vi "WritingDataFile Message Loop.vi"(8 "error in (no error)":errorcluster, 11 "Message Queues":T1) -> (0 "error out":errorcluster)   [LabVIEW 2020, in "WritingDataFile.lvlib"]
uses:
  WritingDataFile.lvlib
  support/Message Queue/All Message Queues.ctl
  support/Message Queue/Message Cluster.ctl
  Modbus/Modbus PLC Data All.ctl
  Modbus/Modbus FVIR Control.ctl
  Modbus/Modbus LDO Control.ctl
  Data to Save.ctl
  <vilib>/Utility/file.llb/Write Delimited Spreadsheet (string).vi
  support/Message Queue/Enqueue Message (Single).vi
  support/Message Queue/Message Queue.lvlib
  Logging/Logging.lvlib
  HeaderForCSV.ctl
  HeaderForCSV_LDO.ctl
panel:
  out "Start time LDO":string
  out "Start time FVIR":string
  out "Numeric":i32
  out "Loop counter":i32
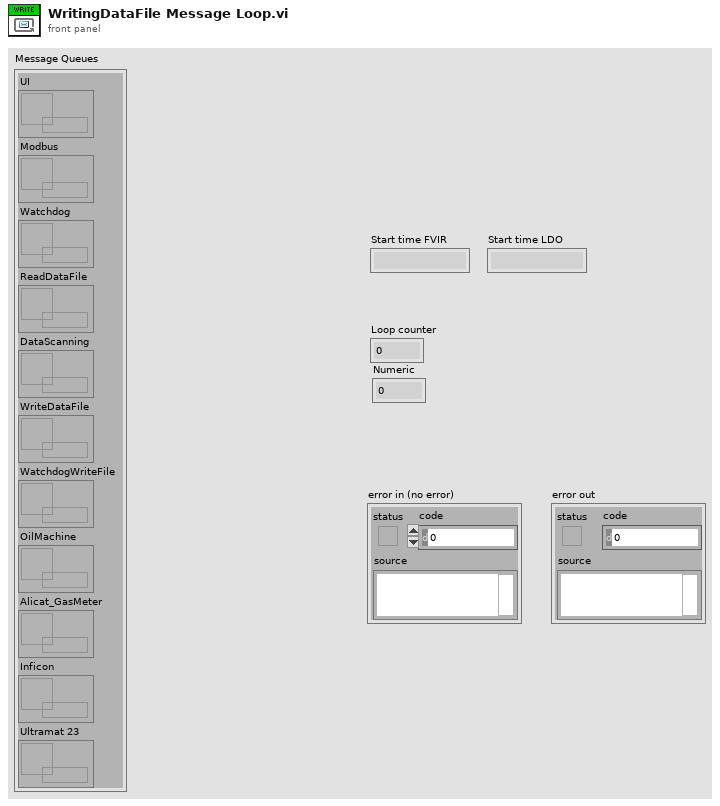
[diagram p1: front panel]
types:
  T1 = typedef "Message Queue.lvlib/All Message Queues.ctl" = cluster{"UI":refnum<queue>, "Modbus":refnum<queue>, "Watchdog":refnum<queue>, "ReadDataFile":refnum<queue>, "DataScanning":refnum<queue>, "WriteDataFile":refnum<queue>, "WatchdogWriteFile":refnum<queue>, "OilMachine":refnum<queue>, "Alicat_GasMeter":refnum<queue>, "Inficon":refnum<queue>, "Ultramat 23":refnum<queue>}
  T2 = typedef "Modbus PLC Data All.ctl" = cluster{"FVIR Data Input":T3, "LDO Control Input":T4, "PLC Input Registers":i16[], "Data to Save":T5}
  T3 = typedef "Modbus FVIR Control.ctl" = cluster{"Spare 15":bool, "Spare 14":bool, "Actuator mannequin is going to Work Pos - FVIR":bool, "Actuator mannequin is going to Home Pos - FVIR":bool, "Test chamber is in sequence - FVIR ":bool, "Water flow DRK375 is open - FVIR":bool, "Gas Solenoid Valve - FVIR":bool, "Water Inlet Valve - FVIR":bool, "Water Outlet Flow Proportional - FVIR":bool, "Start recording data - FVIR":bool, "Actuator spill can is going to Work Pos - FVIR":bool, "Actuator spill can is going to Home Pos - FVIR":bool, "Water Outlet Valve - FVIR":bool, "Can is spilling - FVIR":bool, "Mannequin is moving - FVIR":bool, "FVIR PLC lifebit":bool, "Status for Error - FVIR":string, "Error-FVIR":bool, "Sensors -FVIR":string[][]}
  T4 = typedef "Modbus LDO Control.ctl" = cluster{"LDO PLC Life Bit":bool, "Start recording data - LDO":bool, "Spare 1":bool, "Water Outlet Valve - LDO":bool, "Water Inlet Valve - LDO":bool, "Gas Solenoid Valve - LDO":bool, "Water flow DRK375 is open - LDO":bool, "Test chamber is in sequence - LDO":bool, "Oil spray 0.8cc/min - LDO":bool, "Oil spray 1.1cc/min - LDO":bool, "Oil spray 1.33cc/min - LDO":bool, "Rotary Actuator (ON/OFF) - LDO":bool, "Water Outlet Flow Proportional - LDO":bool, "Conveyor ON/OFF":bool, "Blower ON/OFF":bool, "Spare 4":bool, "Status for error - LDO":string, "Error - LDO":bool, "Sensor Data":string[][], "Thermal Efficiency Rate (GPM)":dbl, "Thermal Efficiency":dbl, "Totalized Flow (Gallons)":dbl, "Counter of oil injections 1.33 cc/min":u16, "Counter of burner cycle":u16, "Counter of oil injections 1.1 cc/min":u16, "Counter of oil injections 0.8 cc/min":u16, "Previous Totalizer (Gallons)":dbl, "Gallon Adder Input":dbl}
  T5 = typedef "Data to Save.ctl" = cluster{"LDO Full Data":string[][], "FVIR Full Data":string[][], "Test Case - FVIR":string, "Test Case - LDO":string}
  T6 = typedef "WritingDataFile.lvlib/HeaderForCSV.ctl" = string[]
  T7 = typedef "WritingDataFile.lvlib/HeaderForCSV_LDO.ctl" = string[]
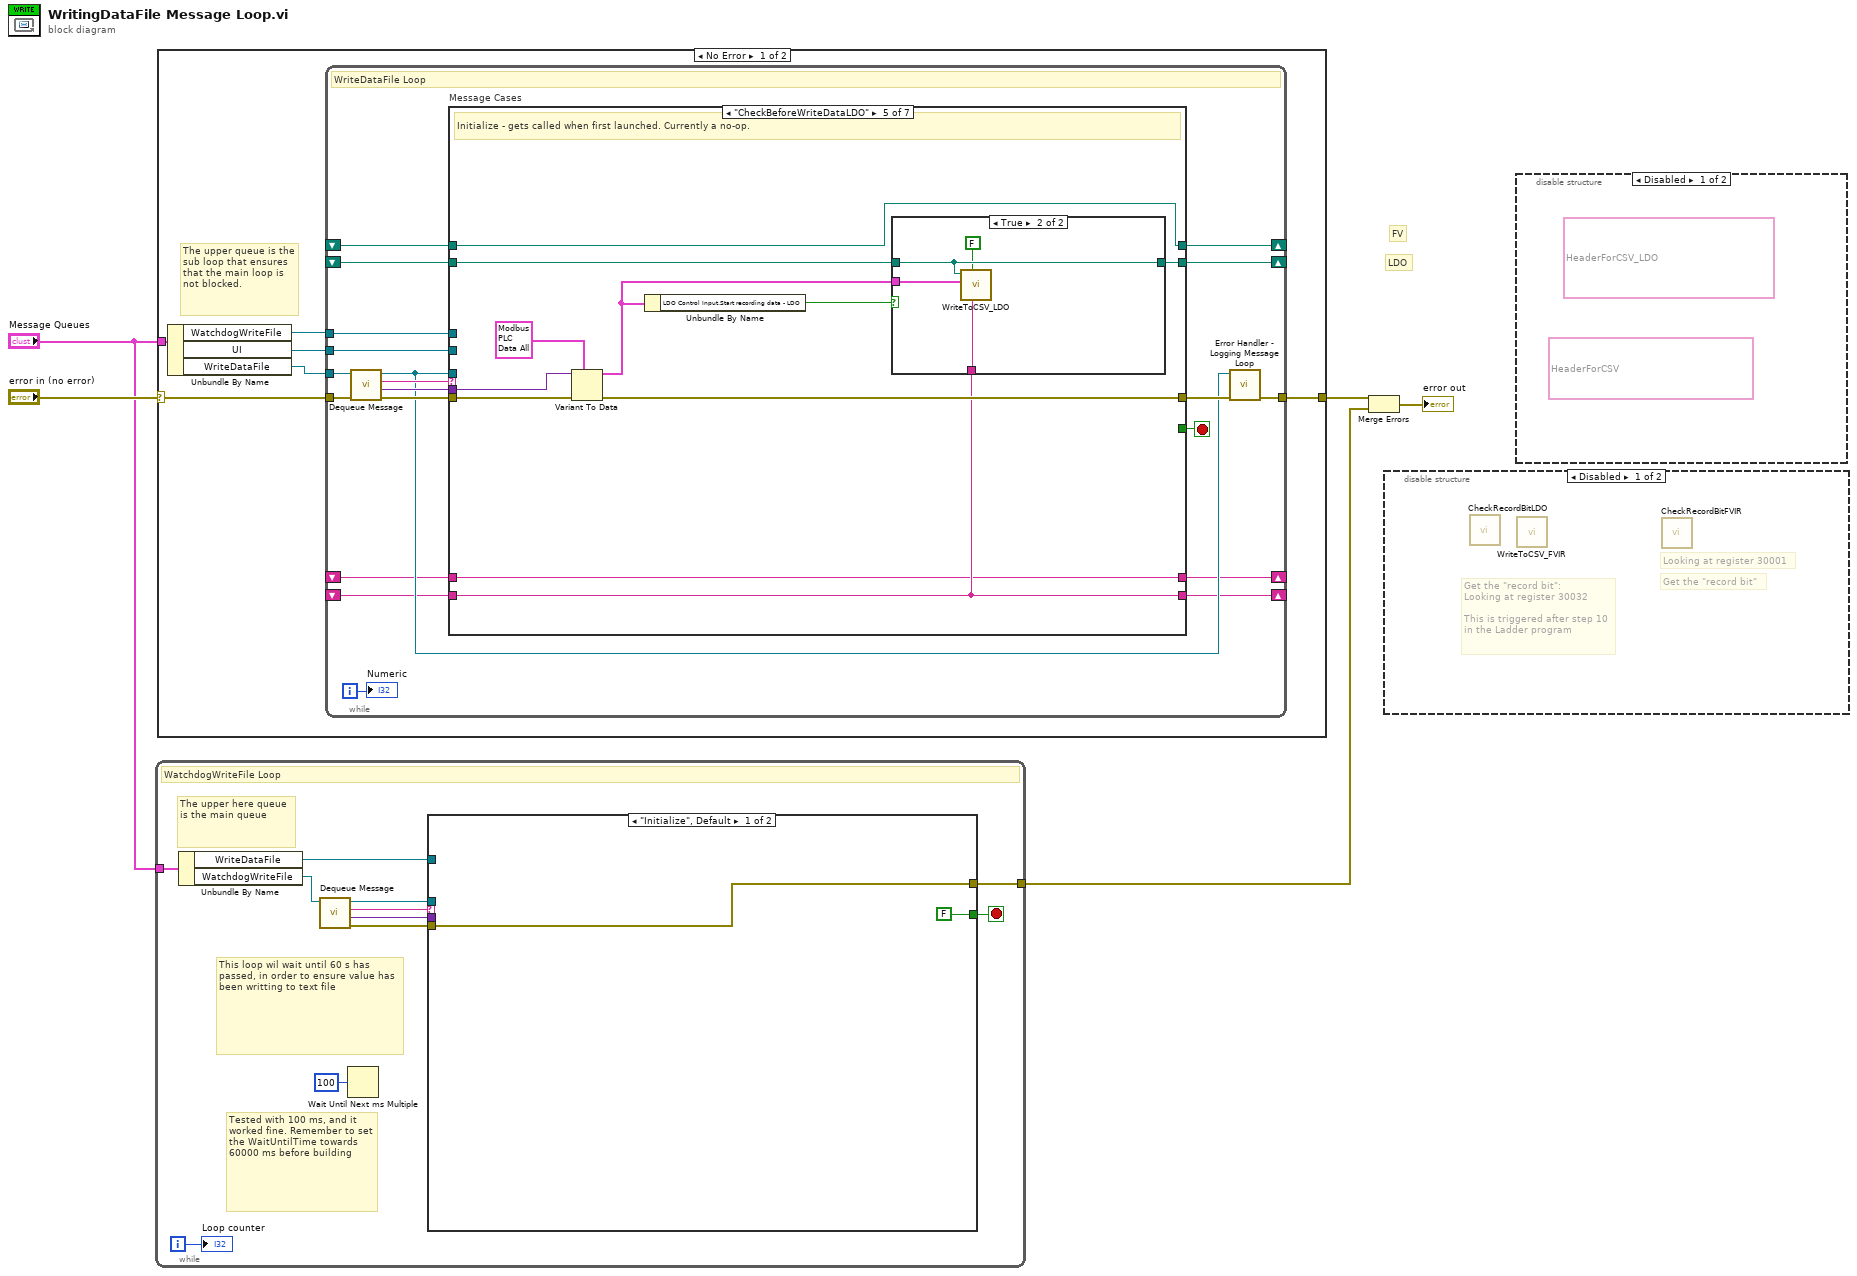
[diagram p0: block diagram]
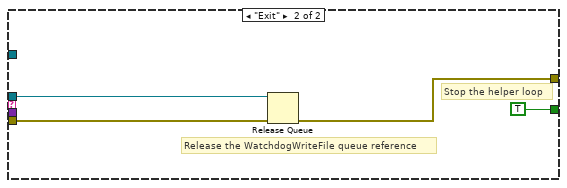
[diagram p4: hidden frame]
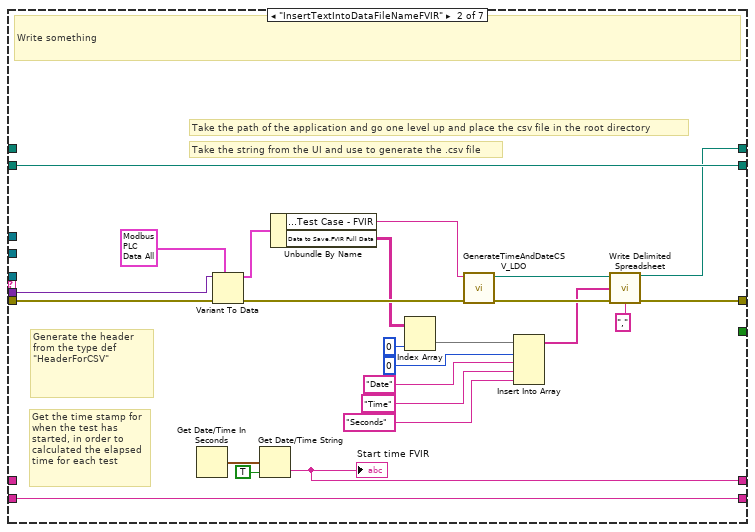
[diagram p6: hidden frame]
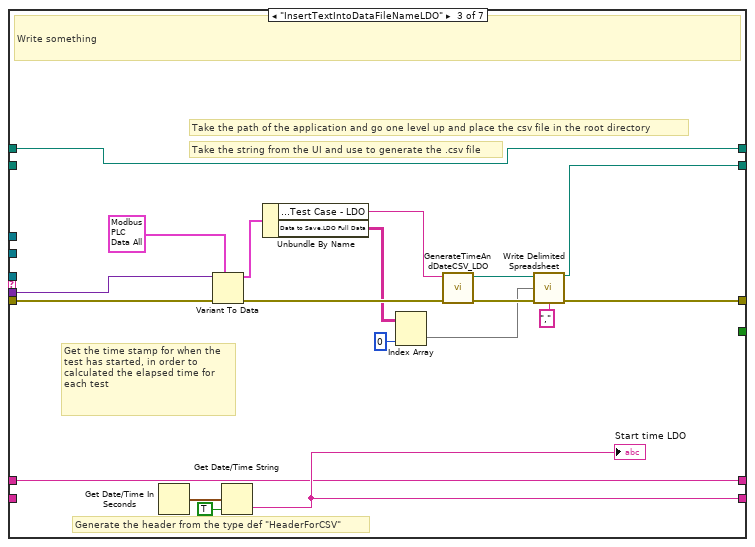
[diagram p7: hidden frame]
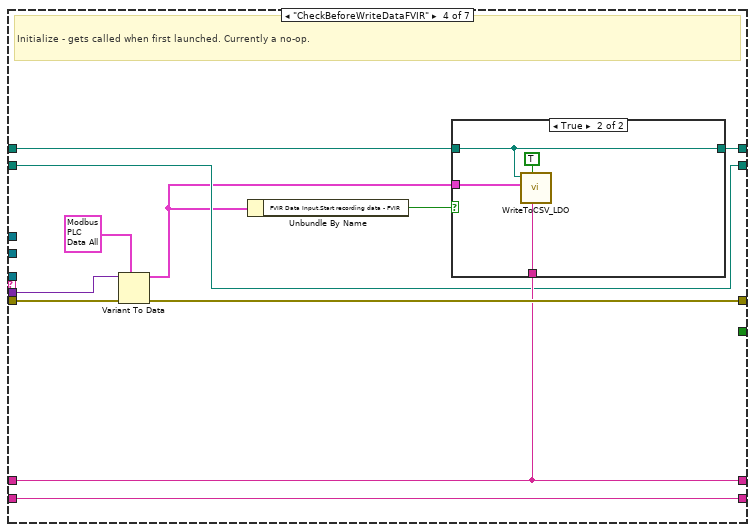
[diagram p8: hidden frame]
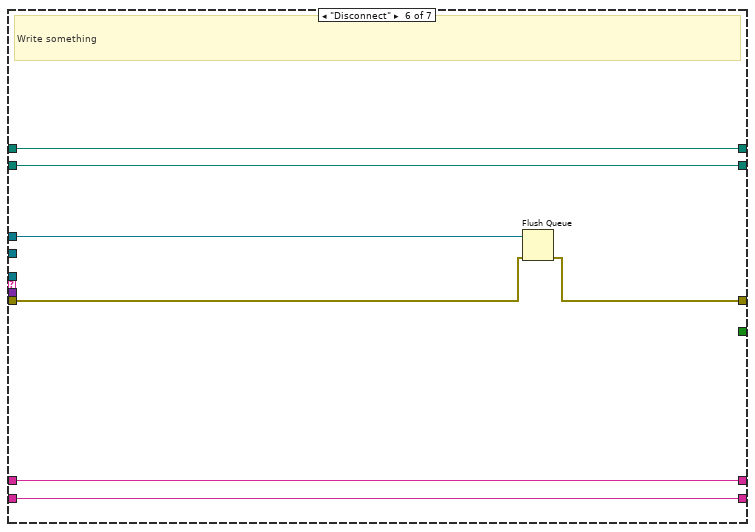
[diagram p11: hidden frame]
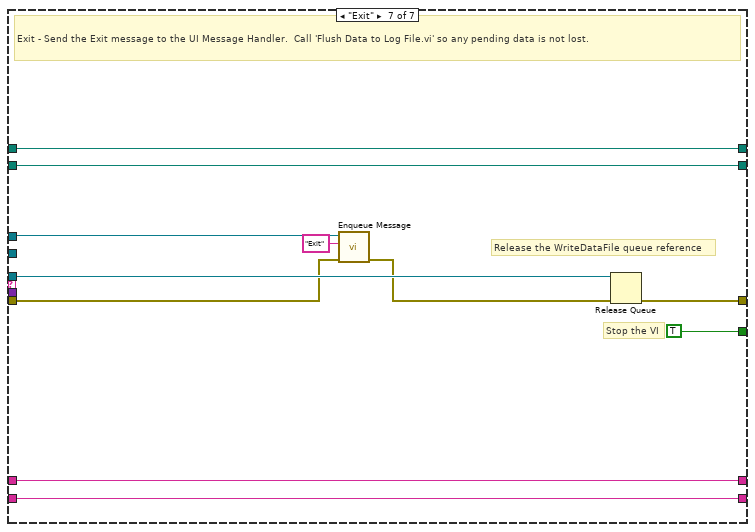
[diagram p12: hidden frame]
diagram:
  # "LDO"
  # "FV"
  n1 = while {
    tunnel: "Message Queues" -> [w16]
    tunnel: [w12] -> w2
    i -> [w7]
    stop <- w13 stop-if-true
    # "Tested with 100 ms, and it worked fine. Remember to set the WaitUntilTime towards 60000 ms before building"
    # "The upper here queue is the main queue"
    # "This loop wil wait until 60 s has passed, in order to ensure value has been writting to text file"
    # "WatchdogWriteFile Loop"
    n2 = Unbundle By Name(w16) -> ("WriteDataFile"=w10:refnum<queue>, "WatchdogWriteFile"=w11:refnum<queue>)
    n3 = call "Dequeue Message.vi"("Message Queue"=w11) -> ("error out"=w14:errorcluster, "Message Data"=w6:variant, "Message"=w15:string, "dup Message Queue"=w9:refnum<queue>)  [unwired: 7 in]
    n4 = Wait Until Next ms Multiple(millisecond multiple=u32 100) -> ()  [unwired: 1 out]
    n5 = case shown="\"Initialize\", Default" w15 {
      tunnel: w14 -> [w18 w22]
      tunnel: [w18 w21] -> w12
      tunnel: [FALSE TRUE] -> w13
      tunnel: w10 -> [_ _]
      tunnel: w9 -> [_ w19]
      tunnel: w6 -> [_ _]
      frame "Initialize", Default {
      }
      frame "Exit" {
        # "Release the WatchdogWriteFile queue reference"
        # "Stop the helper loop"
        n6 = Release Queue(queue=w19, error in (no error)=w22) -> (error out=w21:errorcluster)  [unwired: 1 in, 2 out]
      }
    }
    "Loop counter" <- w7
  }
  n7 = case shown="No Error" "error in (no error)" {
    selector: "error in (no error)" -> [w26 w147]
    tunnel: "Message Queues" -> [w28 _]
    tunnel: [w27 w147] -> w3
    frame No Error {
      # "The upper queue is the sub loop that ensures that the main loop is not blocked."
      n8 = Unbundle By Name(w28) -> ("WatchdogWriteFile"=w25:refnum<queue>, "UI"=w23:refnum<queue>, "WriteDataFile"=w24:refnum<queue>)
      n9 = while {
        tunnel: w24 -> [w43]
        tunnel: w25 -> [w40]
        tunnel: w26 -> [w47]
        tunnel: [w42] -> w27
        tunnel: w23 -> [w38]
        shift-right: [w36] -> _
        shift-left: _ -> [w35]
        shift-right: [w34] -> _
        shift-left: _ -> [w33]
        shift-right: [w32] -> _
        shift-left: _ -> [w31]
        shift-right: [w30] -> _
        shift-left: _ -> [w29]
        i -> [w37]
        stop <- w48 stop-if-true
        # "WriteDataFile Loop"
        n10 = call "Dequeue Message.vi"("error in (no error)"=w47, "Message Queue"=w43) -> ("error out"=w46:errorcluster, "Message Data"=w44:variant, "Message"=w45:string, "dup Message Queue"=w39:refnum<queue>)  [unwired: 6 in]
        n11 = case "Message Cases" shown="\"CheckBeforeWriteDataLDO\"" w45 {
          tunnel: w39 -> [_ _ _ _ _ _ w145]
          tunnel: w46 -> [w53 w77 w96 w107 w123 w134 w140]
          tunnel: [w53 w66 w85 w105 w121 w133 w144] -> w41
          tunnel: [_ _ _ _ _ _ TRUE] -> w48
          tunnel: w44 -> [_ w76 w95 w106 w122 _ _]
          tunnel: w40 -> [_ _ _ _ _ w135 w143]
          tunnel: w38 -> [_ _ _ _ _ _ _]
          tunnel: [w49 w71 w84 w100 w118 w129 w136] -> w36
          tunnel: w35 -> [w49 w71 _ w100 w119 w129 w136]
          tunnel: [w52 w73 w90 w104 w117 w132 w139] -> w34
          tunnel: w33 -> [w52 _ w90 w104 w117 w132 w139]
          tunnel: [w50 w65 w89 w103 w116 w130 w137] -> w32
          tunnel: w31 -> [w50 _ w89 w102 w116 w130 w137]
          tunnel: [w51 w72 w91 w101 w120 w131 w138] -> w30
          tunnel: w29 -> [w51 w72 _ w101 w120 w131 w138]
          frame "Initialize", Default {
            # "Initialize - gets called when first launched. Currently a no-op."
          }
          frame "InsertTextIntoDataFileNameFVIR" {
            # "Get the time stamp for when the test has started, in order to calculated the elapsed time for each test"
            # "Generate the header from the type def \"HeaderForCSV\""
            # "Take the string from the UI and use to generate the .csv file"
            # "Take the path of the application and go one level up and place the csv file in the root directory"
            # "Write something"
            n12 = Get Date/Time In Seconds() -> (seconds since 1Jan1904=w75:timestamp)
            n13 = Variant To Data(error in=w77, type=T2 {"FVIR Data Input"={"Spare 15"=FALSE, "Spare 14"=FALSE, "Actuator mannequin is going to Work Pos - FVIR"=FALSE, "Actuator mannequin is going to Home Pos - FVIR"=FALSE, "Test chamber is in sequence - FVIR "=FALSE, "Water flow DRK375 is open - FVIR"=FALSE, "Gas Solenoid Valve - FVIR"=FALSE, "Water Inlet Valve - FVIR"=FALSE, "Water Outlet Flow Proportional - FVIR"=FALSE, "Start recording data - FVIR"=FALSE, "Actuator spill can is going to Work Pos - FVIR"=FALSE, "Actuator spill can is going to Home Pos - FVIR"=FALSE, "Water Outlet Valve - FVIR"=FALSE, "Can is spilling - FVIR"=FALSE, "Mannequin is moving - FVIR"=FALSE, "FVIR PLC lifebit"=FALSE, "Status for Error - FVIR"="", "Error-FVIR"=FALSE, "Sensors -FVIR"=[]}, "LDO Control Input"={"LDO PLC Life Bit"=FALSE, "Start recording data - LDO"=FALSE, "Spare 1"=FALSE, "Water Outlet Valve - LDO"=FALSE, "Water Inlet Valve - LDO"=FALSE, "Gas Solenoid Valve - LDO"=FALSE, "Water flow DRK375 is open - LDO"=FALSE, "Test chamber is in sequence - LDO"=FALSE, "Oil spray 0.8cc/min - LDO"=FALSE, "Oil spray 1.1cc/min - LDO"=FALSE, "Oil spray 1.33cc/min - LDO"=FALSE, "Rotary Actuator (ON/OFF) - LDO"=FALSE, "Water Outlet Flow Proportional - LDO"=FALSE, "Conveyor ON/OFF"=FALSE, "Blower ON/OFF"=FALSE, "Spare 4"=FALSE, "Status for error - LDO"="", "Error - LDO"=FALSE, "Sensor Data"=[], "Thermal Efficiency Rate (GPM)"=0.0, "Thermal Efficiency"=0.0, "Totalized Flow (Gallons)"=0.0, "Counter of oil injections 1.33 cc/min"=0, "Counter of burner cycle"=0, "Counter of oil injections 1.1 cc/min"=0, "Counter of oil injections 0.8 cc/min"=0, "Previous Totalizer (Gallons)"=0.0, "Gallon Adder Input"=0.0}, "PLC Input Registers"=[], "Data to Save"={"LDO Full Data"=[], "FVIR Full Data"=[], "Test Case - FVIR"="", "Test Case - LDO"=""}} ("PLC Data Out"), Variant=w76) -> (data=w64:T2, error out=w69:errorcluster)
            n14 = Get Date/Time String(seconds (now)=w75, want seconds? (F)=TRUE) -> (time string=w73:string)  [unwired: 1 in, 1 out]
            "Start time FVIR" <- w73
            n15 = Unbundle By Name(w64) -> ("Data to Save.Test Case - FVIR"=w63:string, "Data to Save.FVIR Full Data"=w58:string[][])
            n16 = Index Array(array=w58, index (col)=0 ("disabled index (col)")) -> (element=w62:string[])  [unwired: 1 in]
            n17 = call "GenerateTimeAndDateCSV_LDO.vi"("error in (no error)"=w69, "Test string input"=w63) -> ("error out"=w67:errorcluster, "path for csv file"=w68:path)  [unwired: 8 in]
            n18 = Insert Into Array(array=w62, index=0, new element #1="Date" ("new element/subarray"), new element #2="Time" ("new element/subarray"), new element #3="Seconds" ("new element/subarray")) -> (w57:string[])
            n19 = call-poly <vilib>:"Write Delimited Spreadsheet.vi"("file path (dialog if empty)"=w68, "1D data"=w57, "error in (no error)"=w67, "delimiter (\\t)"="," ("delimiter (\\t)")) -> ("new file path (Not A Path if cancelled)"=w65:path, "error out"=w66:errorcluster)  [unwired: 10 in]
          }
          frame "InsertTextIntoDataFileNameLDO" {
            # "Get the time stamp for when the test has started, in order to calculated the elapsed time for each test"
            # "Generate the header from the type def \"HeaderForCSV\""
            # "Take the string from the UI and use to generate the .csv file"
            # "Take the path of the application and go one level up and place the csv file in the root directory"
            # "Write something"
            n20 = Get Date/Time In Seconds() -> (seconds since 1Jan1904=w94:timestamp)
            n21 = Variant To Data(error in=w96, type=T2 {"FVIR Data Input"={"Spare 15"=FALSE, "Spare 14"=FALSE, "Actuator mannequin is going to Work Pos - FVIR"=FALSE, "Actuator mannequin is going to Home Pos - FVIR"=FALSE, "Test chamber is in sequence - FVIR "=FALSE, "Water flow DRK375 is open - FVIR"=FALSE, "Gas Solenoid Valve - FVIR"=FALSE, "Water Inlet Valve - FVIR"=FALSE, "Water Outlet Flow Proportional - FVIR"=FALSE, "Start recording data - FVIR"=FALSE, "Actuator spill can is going to Work Pos - FVIR"=FALSE, "Actuator spill can is going to Home Pos - FVIR"=FALSE, "Water Outlet Valve - FVIR"=FALSE, "Can is spilling - FVIR"=FALSE, "Mannequin is moving - FVIR"=FALSE, "FVIR PLC lifebit"=FALSE, "Status for Error - FVIR"="", "Error-FVIR"=FALSE, "Sensors -FVIR"=[]}, "LDO Control Input"={"LDO PLC Life Bit"=FALSE, "Start recording data - LDO"=FALSE, "Spare 1"=FALSE, "Water Outlet Valve - LDO"=FALSE, "Water Inlet Valve - LDO"=FALSE, "Gas Solenoid Valve - LDO"=FALSE, "Water flow DRK375 is open - LDO"=FALSE, "Test chamber is in sequence - LDO"=FALSE, "Oil spray 0.8cc/min - LDO"=FALSE, "Oil spray 1.1cc/min - LDO"=FALSE, "Oil spray 1.33cc/min - LDO"=FALSE, "Rotary Actuator (ON/OFF) - LDO"=FALSE, "Water Outlet Flow Proportional - LDO"=FALSE, "Conveyor ON/OFF"=FALSE, "Blower ON/OFF"=FALSE, "Spare 4"=FALSE, "Status for error - LDO"="", "Error - LDO"=FALSE, "Sensor Data"=[], "Thermal Efficiency Rate (GPM)"=0.0, "Thermal Efficiency"=0.0, "Totalized Flow (Gallons)"=0.0, "Counter of oil injections 1.33 cc/min"=0, "Counter of burner cycle"=0, "Counter of oil injections 1.1 cc/min"=0, "Counter of oil injections 0.8 cc/min"=0, "Previous Totalizer (Gallons)"=0.0, "Gallon Adder Input"=0.0}, "PLC Input Registers"=[], "Data to Save"={"LDO Full Data"=[], "FVIR Full Data"=[], "Test Case - FVIR"="", "Test Case - LDO"=""}} ("PLC Data Out"), Variant=w95) -> (data=w83:T2, error out=w87:errorcluster)
            n22 = Get Date/Time String(seconds (now)=w94, want seconds? (F)=TRUE) -> (time string=w91:string)  [unwired: 1 in, 1 out]
            "Start time LDO" <- w91
            n23 = Unbundle By Name(w83) -> ("Data to Save.Test Case - LDO"=w82:string, "Data to Save.LDO Full Data"=w81:string[][])
            n24 = Index Array(array=w81, index (col)=0 ("disabled index (col)")) -> (element=w78:string[])  [unwired: 1 in]
            n25 = call "GenerateTimeAndDateCSV_LDO.vi"("error in (no error)"=w87, "Test string input"=w82) -> ("error out"=w86:errorcluster, "path for csv file"=w92:path)  [unwired: 8 in]
            n26 = call-poly <vilib>:"Write Delimited Spreadsheet.vi"("file path (dialog if empty)"=w92, "1D data"=w78, "error in (no error)"=w86, "delimiter (\\t)"="," ("delimiter (\\t)")) -> ("new file path (Not A Path if cancelled)"=w84:path, "error out"=w85:errorcluster)  [unwired: 10 in]
          }
          frame "CheckBeforeWriteDataFVIR" {
            # "Initialize - gets called when first launched. Currently a no-op."
            n27 = Variant To Data(error in=w107, type=T2 {"FVIR Data Input"={"Spare 15"=FALSE, "Spare 14"=FALSE, "Actuator mannequin is going to Work Pos - FVIR"=FALSE, "Actuator mannequin is going to Home Pos - FVIR"=FALSE, "Test chamber is in sequence - FVIR "=FALSE, "Water flow DRK375 is open - FVIR"=FALSE, "Gas Solenoid Valve - FVIR"=FALSE, "Water Inlet Valve - FVIR"=FALSE, "Water Outlet Flow Proportional - FVIR"=FALSE, "Start recording data - FVIR"=FALSE, "Actuator spill can is going to Work Pos - FVIR"=FALSE, "Actuator spill can is going to Home Pos - FVIR"=FALSE, "Water Outlet Valve - FVIR"=FALSE, "Can is spilling - FVIR"=FALSE, "Mannequin is moving - FVIR"=FALSE, "FVIR PLC lifebit"=FALSE, "Status for Error - FVIR"="", "Error-FVIR"=FALSE, "Sensors -FVIR"=[]}, "LDO Control Input"={"LDO PLC Life Bit"=FALSE, "Start recording data - LDO"=FALSE, "Spare 1"=FALSE, "Water Outlet Valve - LDO"=FALSE, "Water Inlet Valve - LDO"=FALSE, "Gas Solenoid Valve - LDO"=FALSE, "Water flow DRK375 is open - LDO"=FALSE, "Test chamber is in sequence - LDO"=FALSE, "Oil spray 0.8cc/min - LDO"=FALSE, "Oil spray 1.1cc/min - LDO"=FALSE, "Oil spray 1.33cc/min - LDO"=FALSE, "Rotary Actuator (ON/OFF) - LDO"=FALSE, "Water Outlet Flow Proportional - LDO"=FALSE, "Conveyor ON/OFF"=FALSE, "Blower ON/OFF"=FALSE, "Spare 4"=FALSE, "Status for error - LDO"="", "Error - LDO"=FALSE, "Sensor Data"=[], "Thermal Efficiency Rate (GPM)"=0.0, "Thermal Efficiency"=0.0, "Totalized Flow (Gallons)"=0.0, "Counter of oil injections 1.33 cc/min"=0, "Counter of burner cycle"=0, "Counter of oil injections 1.1 cc/min"=0, "Counter of oil injections 0.8 cc/min"=0, "Previous Totalizer (Gallons)"=0.0, "Gallon Adder Input"=0.0}, "PLC Input Registers"=[], "Data to Save"={"LDO Full Data"=[], "FVIR Full Data"=[], "Test Case - FVIR"="", "Test Case - LDO"=""}} ("PLC Data Out"), Variant=w106) -> (data=w98:T2, error out=w105:errorcluster)
            n28 = Unbundle By Name(w98) -> ("FVIR Data Input.Start recording data - FVIR"=w97:bool)
            n29 = case shown="True" w97 {
              tunnel: w98 -> [_ w112]
              tunnel: w104 -> [_ w109]
              tunnel: [w108 w111] -> w103
              tunnel: w102 -> [w108 w111]
              frame False {
              }
              frame True {
                n30 = call "WriteToCSV_LDO.vi"("StartTime"=w109, "FVIR?"=TRUE, "PLC Data Out"=w112, "file path (dialog if empty)"=w111) -> ()  [unwired: 8 in]
              }
            }
          }
          frame "CheckBeforeWriteDataLDO" {
            # "Initialize - gets called when first launched. Currently a no-op."
            n31 = Variant To Data(error in=w123, type=T2 {"FVIR Data Input"={"Spare 15"=FALSE, "Spare 14"=FALSE, "Actuator mannequin is going to Work Pos - FVIR"=FALSE, "Actuator mannequin is going to Home Pos - FVIR"=FALSE, "Test chamber is in sequence - FVIR "=FALSE, "Water flow DRK375 is open - FVIR"=FALSE, "Gas Solenoid Valve - FVIR"=FALSE, "Water Inlet Valve - FVIR"=FALSE, "Water Outlet Flow Proportional - FVIR"=FALSE, "Start recording data - FVIR"=FALSE, "Actuator spill can is going to Work Pos - FVIR"=FALSE, "Actuator spill can is going to Home Pos - FVIR"=FALSE, "Water Outlet Valve - FVIR"=FALSE, "Can is spilling - FVIR"=FALSE, "Mannequin is moving - FVIR"=FALSE, "FVIR PLC lifebit"=FALSE, "Status for Error - FVIR"="", "Error-FVIR"=FALSE, "Sensors -FVIR"=[]}, "LDO Control Input"={"LDO PLC Life Bit"=FALSE, "Start recording data - LDO"=FALSE, "Spare 1"=FALSE, "Water Outlet Valve - LDO"=FALSE, "Water Inlet Valve - LDO"=FALSE, "Gas Solenoid Valve - LDO"=FALSE, "Water flow DRK375 is open - LDO"=FALSE, "Test chamber is in sequence - LDO"=FALSE, "Oil spray 0.8cc/min - LDO"=FALSE, "Oil spray 1.1cc/min - LDO"=FALSE, "Oil spray 1.33cc/min - LDO"=FALSE, "Rotary Actuator (ON/OFF) - LDO"=FALSE, "Water Outlet Flow Proportional - LDO"=FALSE, "Conveyor ON/OFF"=FALSE, "Blower ON/OFF"=FALSE, "Spare 4"=FALSE, "Status for error - LDO"="", "Error - LDO"=FALSE, "Sensor Data"=[], "Thermal Efficiency Rate (GPM)"=0.0, "Thermal Efficiency"=0.0, "Totalized Flow (Gallons)"=0.0, "Counter of oil injections 1.33 cc/min"=0, "Counter of burner cycle"=0, "Counter of oil injections 1.1 cc/min"=0, "Counter of oil injections 0.8 cc/min"=0, "Previous Totalizer (Gallons)"=0.0, "Gallon Adder Input"=0.0}, "PLC Input Registers"=[], "Data to Save"={"LDO Full Data"=[], "FVIR Full Data"=[], "Test Case - FVIR"="", "Test Case - LDO"=""}} ("PLC Data Out"), Variant=w122) -> (data=w114:T2, error out=w121:errorcluster)
            n32 = Unbundle By Name(w114) -> ("LDO Control Input.Start recording data - LDO"=w113:bool)
            n33 = case shown="True" w113 {
              tunnel: w114 -> [_ w126]
              tunnel: w120 -> [_ w127]
              tunnel: w119 -> [w124 w128]
              tunnel: [w124 w128] -> w118
              frame False {
              }
              frame True {
                n34 = call "WriteToCSV_LDO.vi"("StartTime"=w127, "FVIR?"=FALSE, "PLC Data Out"=w126, "file path (dialog if empty)"=w128) -> ()  [unwired: 8 in]
              }
            }
          }
          frame "Disconnect" {
            # "Write something"
            n35 = Flush Queue(queue=w135, error in (no error)=w134) -> (error out=w133:errorcluster)  [unwired: 2 out]
          }
          frame "Exit" {
            # "Release the WriteDataFile queue reference"
            # "Stop the VI"
            # "Exit - Send the Exit message to the UI Message Handler.  Call 'Flush Data to Log File.vi' so any pending data is not lost."
            n36 = call-poly "Enqueue Message.vi"("error in (no error)"=w140, "Message"="Exit", "Message Queue"=w143) -> ("error out"=w141:errorcluster)  [unwired: 7 in, 1 out]
            n37 = Release Queue(queue=w145, error in (no error)=w141) -> (error out=w144:errorcluster)  [unwired: 1 in, 2 out]
          }
        }
        n38 = call "Error Handler - Logging Message Loop.vi"("error in (no error)"=w41, "Message Queue"=w39) -> ("dup error in"=w42:errorcluster)  [unwired: 8 in, 1 out]
        "Numeric" <- w37
      }
    }
    frame Error {
    }
  }
  n39 = Merge Errors(w3, w2) -> (→"error out":errorcluster)
  n40 = disable-structure shown="Disabled" {
    frame Disabled {
      # "Looking at register 30001"
      # "Get the \"record bit\""
      # "Get the \"record bit\":\nLooking at register 30032\n\nThis is triggered after step 10\nin the Ladder program"
      n41 = call "CheckRecordBitLDO.vi"() -> ()  [unwired: 11 in, 1 out]
      n42 = call "WriteToCSV_FVIR.vi"() -> ()  [unwired: 12 in]
      n43 = call "CheckRecordBitFVIR.vi"() -> ()  [unwired: 11 in, 1 out]
    }
    frame Enabled {
    }
  }
  n44 = disable-structure shown="Disabled" {
    frame Disabled {
      (unwired) T6 ["Sample date", "Timestamp", "Starting time time", "Elapsed time seconds", "Register 30001", "Register 30002", "Register 30003", "Register 30004", "Register 30005", "Register 30006", "Register 30007", "Register 30008", "Register 30009", "Register 30010", "Register 30011", "Register 30012", "Register 30013", "Register 30014", "Register 30015", "Register 30016", "Register 30017", "Register 30018", "Register 30019", "Register 30020", "Register 30021", "Register 30022", "Register 30023", "Register 30024", "Register 30025", "Register 30026", "Register 30027", "Register 30028", "Register 30029", "Register 30030", "Register 30031"] ("new element/subarray 2")
      (unwired) T7 ["Sample date", "Timestamp", "Starting time time", "Elapsed time seconds", "Register 30032", "Register 30033", "Register 30034", "Register 30035", "Register 30036", "Register 30037", "Register 30038", "Register 30039", "Register 30040", "Register 30041", "Register 30042", "Register 30043", "Register 30044", "Register 30045", "Register 30046", "Register 30047", "Register 30048", "Register 30049", "Register 30050", "Register 30051", "Register 30052", "Register 30053", "Register 30054", "Register 30055", "Register 30056", "Register 30057"] ("new element/subarray")
    }
    frame Enabled {
    }
  }
